vi "App - analyze RUS V6.vi"() -> ()   [LabVIEW 2015] (continued)
oling_2nd_try/September_2014/091714/39.66500K_500_2500_2.10000V_0.00000T_Sep17-2014__15-02-56_001_091714.bin", "last mod"=timestamp(3493825376 s since 1904-01-01), "file name str"="D:\\Data\\Ultrasound\\LSCO\\LSCO22__130814c\\5_Cooling_2nd_try\\September_2014\\091714\\39.66500K_500_2500_2.10000V_0.00000T_Sep17-2014__15-02-56_001_091714.bin", "mod time(min)"=58230422.93333333, "file format"=enum."binary", "power(V)"=2.1, "Magn Field(T) "=0.0}, {"temperature"=39.59, "temperature str"="39.59000", "file path"=path "D:/Data/Ultrasound/LSCO/LSCO22__130814c/5_Cooling_2nd_try/September_2014/091714/39.59000K_500_2500_2.10000V_0.00000T_Sep17-2014__15-04-15_001_091714.bin", "last mod"=timestamp(3493825455 s since 1904-01-01), "file name str"="D:\\Data\\Ultrasound\\LSCO\\LSCO22__130814c\\5_Cooling_2nd_try\\September_2014\\091714\\39.59000K_500_2500_2.10000V_0.00000T_Sep17-2014__15-04-15_001_091714.bin", "mod time(min)"=58230424.25, "file format"=enum."binary", "power(V)"=2.1, "Magn Field(T) "=0.0}, {"temperature"=39.502, "temperature str"="39.50200", "file path"=path "D:/Data/Ultrasound/LSCO/LSCO22__130814c/5_Cooling_2nd_try/September_2014/091714/39.50200K_500_2500_2.10000V_0.00000T_Sep17-2014__15-05-35_001_091714.bin", "last mod"=timestamp(3493825535 s since 1904-01-01), "file name str"="D:\\Data\\Ultrasound\\LSCO\\LSCO22__130814c\\5_Cooling_2nd_try\\September_2014\\091714\\39.50200K_500_2500_2.10000V_0.00000T_Sep17-2014__15-05-35_001_091714.bin", "mod time(min)"=58230425.583333336, "file format"=enum."binary", "power(V)"=2.1, "Magn Field(T) "=0.0}, {"temperature"=39.427, "temperature str"="39.42700", "file path"=path "D:/Data/Ultrasound/LSCO/LSCO22__130814c/5_Cooling_2nd_try/September_2014/091714/39.42700K_500_2500_2.10000V_0.00000T_Sep17-2014__15-06-54_001_091714.bin", "last mod"=timestamp(3493825614 s since 1904-01-01), "file name str"="D:\\Data\\Ultrasound\\LSCO\\LSCO22__130814c\\5_Cooling_2nd_try\\September_2014\\091714\\39.42700K_500_2500_2.10000V_0.00000T_Sep17-2014__15-06-54_001_091714.bin", "mod time(min)"=58230426.9, "file format"=enum."binary", "power(V)"=2.1, "Magn Field(T) "=0.0}, {"temperature"=39.345, "temperature str"="39.34500", "file path"=path "D:/Data/Ultrasound/LSCO/LSCO22__130814c/5_Cooling_2nd_try/September_2014/091714/39.34500K_500_2500_2.10000V_0.00000T_Sep17-2014__15-08-13_001_091714.bin", "last mod"=timestamp(3493825693 s since 1904-01-01), "file name str"="D:\\Data\\Ultrasound\\LSCO\\LSCO22__130814c\\5_Cooling_2nd_try\\September_2014\\091714\\39.34500K_500_2500_2.10000V_0.00000T_Sep17-2014__15-08-13_001_091714.bin", "mod time(min)"=58230428.21666667, "file format"=enum."binary", "power(V)"=2.1, "Magn Field(T) "=0.0}, {"temperature"=39.266, "temperature str"="39.26600", "file path"=path "D:/Data/Ultrasound/LSCO/LSCO22__130814c/5_Cooling_2nd_try/September_2014/091714/39.26600K_500_2500_2.10000V_0.00000T_Sep17-2014__15-09-33_001_091714.bin", "last mod"=timestamp(3493825773 s since 1904-01-01), "file name str"="D:\\Data\\Ultrasound\\LSCO\\LSCO22__130814c\\5_Cooling_2nd_try\\September_2014\\091714\\39.26600K_500_2500_2.10000V_0.00000T_Sep17-2014__15-09-33_001_091714.bin", "mod time(min)"=58230429.55, "file format"=enum."binary", "power(V)"=2.1, "Magn Field(T) "=0.0}, {"temperature"=39.182, "temperature str"="39.18200", "file path"=path "D:/Data/Ultrasound/LSCO/LSCO22__130814c/5_Cooling_2nd_try/September_2014/091714/39.18200K_500_2500_2.10000V_0.00000T_Sep17-2014__15-10-52_001_091714.bin", "last mod"=timestamp(3493825852 s since 1904-01-01), "file name str"="D:\\Data\\Ultrasound\\LSCO\\LSCO22__130814c\\5_Cooling_2nd_try\\September_2014\\091714\\39.18200K_500_2500_2.10000V_0.00000T_Sep17-2014__15-10-52_001_091714.bin", "mod time(min)"=58230430.86666667, "file format"=enum."binary", "power(V)"=2.1, "Magn Field(T) "=0.0}, {"temperature"=39.106, "temperature str"="39.10600", "file path"=path "D:/Data/Ultrasound/LSCO/LSCO22__130814c/5_Cooling_2nd_try/September_2014/091714/39.10600K_500_2500_2.10000V_0.00000T_Sep17-2014__15-12-11_001_091714.bin", "last mod"=timestamp(3493825931 s since 1904-01-01), "file name str"="D:\\Data\\Ultrasound\\LSCO\\LSCO22__130814c\\5_Cooling_2nd_try\\September_2014\\091714\\39.10600K_500_2500_2.10000V_0.00000T_Sep17-2014__15-12-11_001_091714.bin", "mod time(min)"=58230432.18333333, "file format"=enum."binary", "power(V)"=2.1, "Magn Field(T) "=0.0}, {"temperature"=39.022, "temperature str"="39.02200", "file path"=path "D:/Data/Ultrasound/LSCO/LSCO22__130814c/5_Cooling_2nd_try/September_2014/091714/39.02200K_500_2500_2.10000V_0.00000T_Sep17-2014__15-13-31_001_091714.bin", "last mod"=timestamp(3493826011 s since 1904-01-01), "file name str"="D:\\Data\\Ultrasound\\LSCO\\LSCO22__130814c\\5_Cooling_2nd_try\\September_2014\\091714\\39.02200K_500_2500_2.10000V_0.00000T_Sep17-2014__15-13-31_001_091714.bin", "mod time(min)"=58230433.516666666, "file format"=enum."binary", "power(V)"=2.1, "Magn Field(T) "=0.0}, {"temperature"=38.943, "temperature str"="38.94300", "file path"=path "D:/Data/Ultrasound/LSCO/LSCO22__130814c/5_Cooling_2nd_try/September_2014/091714/38.94300K_500_2500_2.10000V_0.00000T_Sep17-2014__15-14-50_001_091714.bin", "last mod"=timestamp(3493826090 s since 1904-01-01), "file name str"="D:\\Data\\Ultrasound\\LSCO\\LSCO22__130814c\\5_Cooling_2nd_try\\September_2014\\091714\\38.94300K_500_2500_2.10000V_0.00000T_Sep17-2014__15-14-50_001_091714.bin", "mod time(min)"=58230434.833333336, "file format"=enum."binary", "power(V)"=2.1, "Magn Field(T) "=0.0}, {"temperature"=38.864, "temperature str"="38.86400", "file path"=path "D:/Data/Ultrasound/LSCO/LSCO22__130814c/5_Cooling_2nd_try/September_2014/091714/38.86400K_500_2500_2.10000V_0.00000T_Sep17-2014__15-16-10_001_091714.bin", "last mod"=timestamp(3493826170 s since 1904-01-01), "file name str"="D:\\Data\\Ultrasound\\LSCO\\LSCO22__130814c\\5_Cooling_2nd_try\\September_2014\\091714\\38.86400K_500_2500_2.10000V_0.00000T_Sep17-2014__15-16-10_001_091714.bin", "mod time(min)"=58230436.166666664, "file format"=enum."binary", "power(V)"=2.1, "Magn Field(T) "=0.0}, {"temperature"=38.78, "temperature str"="38.78000", "file path"=path "D:/Data/Ultrasound/LSCO/LSCO22__130814c/5_Cooling_2nd_try/September_2014/091714/38.78000K_500_2500_2.10000V_0.00000T_Sep17-2014__15-17-29_001_091714.bin", "last mod"=timestamp(3493826249 s since 1904-01-01), "file name str"="D:\\Data\\Ultrasound\\LSCO\\LSCO22__130814c\\5_Cooling_2nd_try\\September_2014\\091714\\38.78000K_500_2500_2.10000V_0.00000T_Sep17-2014__15-17-29_001_091714.bin", "mod time(min)"=58230437.483333334, "file format"=enum."binary", "power(V)"=2.1, "Magn Field(T) "=0.0}, {"temperature"=38.695, "temperature str"="38.69500", "file path"=path "D:/Data/Ultrasound/LSCO/LSCO22__130814c/5_Cooling_2nd_try/September_2014/091714/38.69500K_500_2500_2.10000V_0.00000T_Sep17-2014__15-18-49_001_091714.bin", "last mod"=timestamp(3493826329 s since 1904-01-01), "file name str"="D:\\Data\\Ultrasound\\LSCO\\LSCO22__130814c\\5_Cooling_2nd_try\\September_2014\\091714\\38.69500K_500_2500_2.10000V_0.00000T_Sep17-2014__15-18-49_001_091714.bin", "mod time(min)"=58230438.81666667, "file format"=enum."binary", "power(V)"=2.1, "Magn Field(T) "=0.0}, {"temperature"=38.618, "temperature str"="38.61800", "file path"=path "D:/Data/Ultrasound/LSCO/LSCO22__130814c/5_Cooling_2nd_try/September_2014/091714/38.61800K_500_2500_2.10000V_0.00000T_Sep17-2014__15-20-08_001_091714.bin", "last mod"=timestamp(3493826408 s since 1904-01-01), "file name str"="D:\\Data\\Ultrasound\\LSCO\\LSCO22__130814c\\5_Cooling_2nd_try\\September_2014\\091714\\38.61800K_500_2500_2.10000V_0.00000T_Sep17-2014__15-20-08_001_091714.bin", "mod time(min)"=58230440.13333333, "file format"=enum."binary", "power(V)"=2.1, "Magn Field(T) "=0.0}, {"temperature"=38.531, "temperature str"="38.53100", "file path"=path "D:/Data/Ultrasound/LSCO/LSCO22__130814c/5_Cooling_2nd_try/September_2014/091714/38.53100K_500_2500_2.10000V_0.00000T_Sep17-2014__15-21-27_001_091714.bin", "last mod"=timestamp(3493826487 s since 1904-01-01), "file name str"="D:\\Data\\Ultrasound\\LSCO\\LSCO22__130814c\\5_Cooling_2nd_try\\September_2014\\091714\\38.53100K_500_2500_2.10000V_0.00000T_Sep17-2014__15-21-27_001_091714.bin", "mod time(min)"=58230441.45, "file format"=enum."binary", "power(V)"=2.1, "Magn Field(T) "=0.0}, {"temperature"=38.455, "temperature str"="38.45500", "file path"=path "D:/Data/Ultrasound/LSCO/LSCO22__130814c/5_Cooling_2nd_try/September_2014/091714/38.45500K_500_2500_2.10000V_0.00000T_Sep17-2014__15-22-47_001_091714.bin", "last mod"=timestamp(3493826567 s since 1904-01-01), "file name str"="D:\\Data\\Ultrasound\\LSCO\\LSCO22__130814c\\5_Cooling_2nd_try\\September_2014\\091714\\38.45500K_500_2500_2.10000V_0.00000T_Sep17-2014__15-22-47_001_091714.bin", "mod time(min)"=58230442.78333333, "file format"=enum."binary", "power(V)"=2.1, "Magn Field(T) "=0.0}, {"temperature"=38.37, "temperature str"="38.37000", "file path"=path "D:/Data/Ultrasound/LSCO/LSCO22__130814c/5_Cooling_2nd_try/September_2014/091714/38.37000K_500_2500_2.10000V_0.00000T_Sep17-2014__15-24-06_001_091714.bin", "last mod"=timestamp(3493826646 s since 1904-01-01), "file name str"="D:\\Data\\Ultrasound\\LSCO\\LSCO22__130814c\\5_Cooling_2nd_try\\September_2014\\091714\\38.37000K_500_2500_2.10000V_0.00000T_Sep17-2014__15-24-06_001_091714.bin", "mod time(min)"=58230444.1, "file format"=enum."binary", "power(V)"=2.1, "Magn Field(T) "=0.0}, {"temperature"=38.286, "temperature str"="38.28600", "file path"=path "D:/Data/Ultrasound/LSCO/LSCO22__130814c/5_Cooling_2nd_try/September_2014/091714/38.28600K_500_2500_2.10000V_0.00000T_Sep17-2014__15-25-25_001_091714.bin", "last mod"=timestamp(3493826725 s since 1904-01-01), "file name str"="D:\\Data\\Ultrasound\\LSCO\\LSCO22__130814c\\5_Cooling_2nd_try\\September_2014\\091714\\38.28600K_500_2500_2.10000V_0.00000T_Sep17-2014__15-25-25_001_091714.bin", "mod time(min)"=58230445.416666664, "file format"=enum."binary", "power(V)"=2.1, "Magn Field(T) "=0.0}, {"temperature"=38.203, "temperature str"="38.20300", "file path"=path "D:/Data/Ultrasound/LSCO/LSCO22__130814c/5_Cooling_2nd_try/September_2014/091714/38.20300K_500_2500_2.10000V_0.00000T_Sep17-2014__15-26-45_001_091714.bin", "last mod"=timestamp(3493826805 s since 1904-01-01), "file name str"="D:\\Data\\Ultrasound\\LSCO\\LSCO22__130814c\\5_Cooling_2nd_try\\September_2014\\091714\\38.20300K_500_2500_2.10000V_0.00000T_Sep17-2014__15-26-45_001_091714.bin", "mod time(min)"=58230446.75, "file format"=enum."binary", "power(V)"=2.1, "Magn Field(T) "=0.0}, {"temperature"=38.122, "temperature str"="38.12200", "file path"=path "D:/Data/Ultrasound/LSCO/LSCO22__130814c/5_Cooling_2nd_try/September_2014/091714/38.12200K_500_2500_2.10000V_0.00000T_Sep17-2014__15-28-04_001_091714.bin", "last mod"=timestamp(3493826884 s since 1904-01-01), "file name str"="D:\\Data\\Ultrasound\\LSCO\\LSCO22__130814c\\5_Cooling_2nd_try\\September_2014\\091714\\38.12200K_500_2500_2.10000V_0.00000T_Sep17-2014__15-28-04_001_091714.bin", "mod time(min)"=58230448.06666667, "file format"=enum."binary", "power(V)"=2.1, "Magn Field(T) "=0.0}, {"temperature"=38.042, "temperature str"="38.04200", "file path"=path "D:/Data/Ultrasound/LSCO/LSCO22__130814c/5_Cooling_2nd_try/September_2014/091714/38.04200K_500_2500_2.10000V_0.00000T_Sep17-2014__15-29-24_001_091714.bin", "last mod"=timestamp(3493826964 s since 1904-01-01), "file name str"="D:\\Data\\Ultrasound\\LSCO\\LSCO22__130814c\\5_Cooling_2nd_try\\September_2014\\091714\\38.04200K_500_2500_2.10000V_0.00000T_Sep17-2014__15-29-24_001_091714.bin", "mod time(min)"=58230449.4, "file format"=enum."binary", "power(V)"=2.1, "Magn Field(T) "=0.0}, {"temperature"=37.958, "temperature str"="37.95800", "file path"=path "D:/Data/Ultrasound/LSCO/LSCO22__130814c/5_Cooling_2nd_try/September_2014/091714/37.95800K_500_2500_2.10000V_0.00000T_Sep17-2014__15-30-43_001_091714.bin", "last mod"=timestamp(3493827043 s since 1904-01-01), "file name str"="D:\\Data\\Ultrasound\\LSCO\\LSCO22__130814c\\5_Cooling_2nd_try\\September_2014\\091714\\37.95800K_500_2500_2.10000V_0.00000T_Sep17-2014__15-30-43_001_091714.bin", "mod time(min)"=58230450.71666667, "file format"=enum."binary", "power(V)"=2.1, "Magn Field(T) "=0.0}, {"temperature"=37.876, "temperature str"="37.87600", "file path"=path "D:/Data/Ultrasound/LSCO/LSCO22__130814c/5_Cooling_2nd_try/September_2014/091714/37.87600K_500_2500_2.10000V_0.00000T_Sep17-2014__15-32-02_001_091714.bin", "last mod"=timestamp(3493827122 s since 1904-01-01), "file name str"="D:\\Data\\Ultrasound\\LSCO\\LSCO22__130814c\\5_Cooling_2nd_try\\September_2014\\091714\\37.87600K_500_2500_2.10000V_0.00000T_Sep17-2014__15-32-02_001_091714.bin", "mod time(min)"=58230452.03333333, "file format"=enum."binary", "power(V)"=2.1, "Magn Field(T) "=0.0}, {"temperature"=37.797, "temperature str"="37.79700", "file path"=path "D:/Data/Ultrasound/LSCO/LSCO22__130814c/5_Cooling_2nd_try/September_2014/091714/37.79700K_500_2500_2.10000V_0.00000T_Sep17-2014__15-33-22_001_091714.bin", "last mod"=timestamp(3493827202 s since 1904-01-01), "file name str"="D:\\Data\\Ultrasound\\LSCO\\LSCO22__130814c\\5_Cooling_2nd_try\\September_2014\\091714\\37.79700K_500_2500_2.10000V_0.00000T_Sep17-2014__15-33-22_001_091714.bin", "mod time(min)"=58230453.36666667, "file format"=enum."binary", "power(V)"=2.1, "Magn Field(T) "=0.0}, {"temperature"=37.711, "temperature str"="37.71100", "file path"=path "D:/Data/Ultrasound/LSCO/LSCO22__130814c/5_Cooling_2nd_try/September_2014/091714/37.71100K_500_2500_2.10000V_0.00000T_Sep17-2014__15-34-41_001_091714.bin", "last mod"=timestamp(3493827281 s since 1904-01-01), "file name str"="D:\\Data\\Ultrasound\\LSCO\\LSCO22__130814c\\5_Cooling_2nd_try\\September_2014\\091714\\37.71100K_500_2500_2.10000V_0.00000T_Sep17-2014__15-34-41_001_091714.bin", "mod time(min)"=58230454.68333333, "file format"=enum."binary", "power(V)"=2.1, "Magn Field(T) "=0.0}, {"temperature"=37.627, "temperature str"="37.62700", "file path"=path "D:/Data/Ultrasound/LSCO/LSCO22__130814c/5_Cooling_2nd_try/September_2014/091714/37.62700K_500_2500_2.10000V_0.00000T_Sep17-2014__15-36-00_001_091714.bin", "last mod"=timestamp(3493827360 s since 1904-01-01), "file name str"="D:\\Data\\Ultrasound\\LSCO\\LSCO22__130814c\\5_Cooling_2nd_try\\September_2014\\091714\\37.62700K_500_2500_2.10000V_0.00000T_Sep17-2014__15-36-00_001_091714.bin", "mod time(min)"=58230456.0, "file format"=enum."binary", "power(V)"=2.1, "Magn Field(T) "=0.0}, {"temperature"=37.544, "temperature str"="37.54400", "file path"=path "D:/Data/Ultrasound/LSCO/LSCO22__130814c/5_Cooling_2nd_try/September_2014/091714/37.54400K_500_2500_2.10000V_0.00000T_Sep17-2014__15-37-20_001_091714.bin", "last mod"=timestamp(3493827440 s since 1904-01-01), "file name str"="D:\\Data\\Ultrasound\\LSCO\\LSCO22__130814c\\5_Cooling_2nd_try\\September_2014\\091714\\37.54400K_500_2500_2.10000V_0.00000T_Sep17-2014__15-37-20_001_091714.bin", "mod time(min)"=58230457.333333336, "file format"=enum."binary", "power(V)"=2.1, "Magn Field(T) "=0.0}, {"temperature"=37.459, "temperature str"="37.45900", "file path"=path "D:/Data/Ultrasound/LSCO/LSCO22__130814c/5_Cooling_2nd_try/September_2014/091714/37.45900K_500_2500_2.10000V_0.00000T_Sep17-2014__15-38-39_001_091714.bin", "last mod"=timestamp(3493827519 s since 1904-01-01), "file name str"="D:\\Data\\Ultrasound\\LSCO\\LSCO22__130814c\\5_Cooling_2nd_try\\September_2014\\091714\\37.45900K_500_2500_2.10000V_0.00000T_Sep17-2014__15-38-39_001_091714.bin", "mod time(min)"=58230458.65, "file format"=enum."binary", "power(V)"=2.1, "Magn Field(T) "=0.0}, {"temperature"=37.378, "temperature str"="37.37800", "file path"=path "D:/Data/Ultrasound/LSCO/LSCO22__130814c/5_Cooling_2nd_try/September_2014/091714/37.37800K_500_2500_2.10000V_0.00000T_Sep17-2014__15-39-59_001_091714.bin", "last mod"=timestamp(3493827599 s since 1904-01-01), "file name str"="D:\\Data\\Ultrasound\\LSCO\\LSCO22__130814c\\5_Cooling_2nd_try\\September_2014\\091714\\37.37800K_500_2500_2.10000V_0.00000T_Sep17-2014__15-39-59_001_091714.bin", "mod time(min)"=58230459.983333334, "file format"=enum."binary", "power(V)"=2.1, "Magn Field(T) "=0.0}, {"temperature"=37.297, "temperature str"="37.29700", "file path"=path "D:/Data/Ultrasound/LSCO/LSCO22__130814c/5_Cooling_2nd_try/September_2014/091714/37.29700K_500_2500_2.10000V_0.00000T_Sep17-2014__15-41-18_001_091714.bin", "last mod"=timestamp(3493827678 s since 1904-01-01), "file name str"="D:\\Data\\Ultrasound\\LSCO\\LSCO22__130814c\\5_Cooling_2nd_try\\September_2014\\091714\\37.29700K_500_2500_2.10000V_0.00000T_Sep17-2014__15-41-18_001_091714.bin", "mod time(min)"=58230461.3, "file format"=enum."binary", "power(V)"=2.1, "Magn Field(T) "=0.0}, {"temperature"=37.206, "temperature str"="37.20600", "file path"=path "D:/Data/Ultrasound/LSCO/LSCO22__130814c/5_Cooling_2nd_try/September_2014/091714/37.20600K_500_2500_2.10000V_0.00000T_Sep17-2014__15-42-37_001_091714.bin", "last mod"=timestamp(3493827757 s since 1904-01-01), "file name str"="D:\\Data\\Ultrasound\\LSCO\\LSCO22__130814c\\5_Cooling_2nd_try\\September_2014\\091714\\37.20600K_500_2500_2.10000V_0.00000T_Sep17-2014__15-42-37_001_091714.bin", "mod time(min)"=58230462.61666667, "file format"=enum."binary", "power(V)"=2.1, "Magn Field(T) "=0.0}, {"temperature"=37.129, "temperature str"="37.12900", "file path"=path "D:/Data/Ultrasound/LSCO/LSCO22__130814c/5_Cooling_2nd_try/September_2014/091714/37.12900K_500_2500_2.10000V_0.00000T_Sep17-2014__15-43-57_001_091714.bin", "last mod"=timestamp(3493827837 s since 1904-01-01), "file name str"="D:\\Data\\Ultrasound\\LSCO\\LSCO22__130814c\\5_Cooling_2nd_try\\September_2014\\091714\\37.12900K_500_2500_2.10000V_0.00000T_Sep17-2014__15-43-57_001_091714.bin", "mod time(min)"=58230463.95, "file format"=enum."binary", "power(V)"=2.1, "Magn Field(T) "=0.0}, {"temperature"=37.038, "temperature str"="37.03800", "file path"=path "D:/Data/Ultrasound/LSCO/LSCO22__130814c/5_Cooling_2nd_try/September_2014/091714/37.03800K_500_2500_2.10000V_0.00000T_Sep17-2014__15-45-16_001_091714.bin", "last mod"=timestamp(3493827916 s since 1904-01-01), "file name str"="D:\\Data\\Ultrasound\\LSCO\\LSCO22__130814c\\5_Cooling_2nd_try\\September_2014\\091714\\37.03800K_500_2500_2.10000V_0.00000T_Sep17-2014__15-45-16_001_091714.bin", "mod time(min)"=58230465.266666666, "file format"=enum."binary", "power(V)"=2.1, "Magn Field(T) "=0.0}, {"temperature"=36.964, "temperature str"="36.96400", "file path"=path "D:/Data/Ultrasound/LSCO/LSCO22__130814c/5_Cooling_2nd_try/September_2014/091714/36.96400K_500_2500_2.10000V_0.00000T_Sep17-2014__15-46-35_001_091714.bin", "last mod"=timestamp(3493827995 s since 1904-01-01), "file name str"="D:\\Data\\Ultrasound\\LSCO\\LSCO22__130814c\\5_Cooling_2nd_try\\September_2014\\091714\\36.96400K_500_2500_2.10000V_0.00000T_Sep17-2014__15-46-35_001_091714.bin", "mod time(min)"=58230466.583333336, "file format"=enum."binary", "power(V)"=2.1, "Magn Field(T) "=0.0}, {"temperature"=36.875, "temperature str"="36.87500", "file path"=path "D:/Data/Ultrasound/LSCO/LSCO22__130814c/5_Cooling_2nd_try/September_2014/091714/36.87500K_500_2500_2.10000V_0.00000T_Sep17-2014__15-47-55_001_091714.bin", "last mod"=timestamp(3493828075 s since 1904-01-01), "file name str"="D:\\Data\\Ultrasound\\LSCO\\LSCO22__130814c\\5_Cooling_2nd_try\\September_2014\\091714\\36.87500K_500_2500_2.10000V_0.00000T_Sep17-2014__15-47-55_001_091714.bin", "mod time(min)"=58230467.916666664, "file format"=enum."binary", "power(V)"=2.1, "Magn Field(T) "=0.0}, {"temperature"=36.787, "temperature str"="36.78700", "file path"=path "D:/Data/Ultrasound/LSCO/LSCO22__130814c/5_Cooling_2nd_try/September_2014/091714/36.78700K_500_2500_2.10000V_0.00000T_Sep17-2014__15-49-14_001_091714.bin", "last mod"=timestamp(3493828154 s since 1904-01-01), "file name str"="D:\\Data\\Ultrasound\\LSCO\\LSCO22__130814c\\5_Cooling_2nd_try\\September_2014\\091714\\36.78700K_500_2500_2.10000V_0.00000T_Sep17-2014__15-49-14_001_091714.bin", "mod time(min)"=58230469.233333334, "file format"=enum."binary", "power(V)"=2.1, "Magn Field(T) "=0.0}, {"temperature"=36.71, "temperature str"="36.71000", "file path"=path "D:/Data/Ultrasound/LSCO/LSCO22__130814c/5_Cooling_2nd_try/September_2014/091714/36.71000K_500_2500_2.10000V_0.00000T_Sep17-2014__15-50-34_001_091714.bin", "last mod"=timestamp(3493828234 s since 1904-01-01), "file name str"="D:\\Data\\Ultrasound\\LSCO\\LSCO22__130814c\\5_Cooling_2nd_try\\September_2014\\091714\\36.71000K_500_2500_2.10000V_0.00000T_Sep17-2014__15-50-34_001_091714.bin", "mod time(min)"=58230470.56666667, "file format"=enum."binary", "power(V)"=2.1, "Magn Field(T) "=0.0}, {"temperature"=36.616, "temperature str"="36.61600", "file path"=path "D:/Data/Ultrasound/LSCO/LSCO22__130814c/5_Cooling_2nd_try/September_2014/091714/36.61600K_500_2500_2.10000V_0.00000T_Sep17-2014__15-51-53_001_091714.bin", "last mod"=timestamp(3493828313 s since 1904-01-01), "file name str"="D:\\Data\\Ultrasound\\LSCO\\LSCO22__130814c\\5_Cooling_2nd_try\\September_2014\\091714\\36.61600K_500_2500_2.10000V_0.00000T_Sep17-2014__15-51-53_001_091714.bin", "mod time(min)"=58230471.88333333, "file format"=enum."binary", "power(V)"=2.1, "Magn Field(T) "=0.0}, {"temperature"=36.538, "temperature str"="36.53800", "file path"=path "D:/Data/Ultrasound/LSCO/LSCO22__130814c/5_Cooling_2nd_try/September_2014/091714/36.53800K_500_2500_2.10000V_0.00000T_Sep17-2014__15-53-12_001_091714.bin", "last mod"=timestamp(3493828392 s since 1904-01-01), "file name str"="D:\\Data\\Ultrasound\\LSCO\\LSCO22__130814c\\5_Cooling_2nd_try\\September_2014\\091714\\36.53800K_500_2500_2.10000V_0.00000T_Sep17-2014__15-53-12_001_091714.bin", "mod time(min)"=58230473.2, "file format"=enum."binary", "power(V)"=2.1, "Magn Field(T) "=0.0}, {"temperature"=36.457, "temperature str"="36.45700", "file path"=path "D:/Data/Ultrasound/LSCO/LSCO22__130814c/5_Cooling_2nd_try/September_2014/091714/36.45700K_500_2500_2.10000V_0.00000T_Sep17-2014__15-54-32_001_091714.bin", "last mod"=timestamp(3493828472 s since 1904-01-01), "file name str"="D:\\Data\\Ultrasound\\LSCO\\LSCO22__130814c\\5_Cooling_2nd_try\\September_2014\\091714\\36.45700K_500_2500_2.10000V_0.00000T_Sep17-2014__15-54-32_001_091714.bin", "mod time(min)"=58230474.53333333, "file format"=enum."binary", "power(V)"=2.1, "Magn Field(T) "=0.0}, {"temperature"=36.365, "temperature str"="36.36500", "file path"=path "D:/Data/Ultrasound/LSCO/LSCO22__130814c/5_Cooling_2nd_try/September_2014/091714/36.36500K_500_2500_2.10000V_0.00000T_Sep17-2014__15-55-51_001_091714.bin", "last mod"=timestamp(3493828551 s since 1904-01-01), "file name str"="D:\\Data\\Ultrasound\\LSCO\\LSCO22__130814c\\5_Cooling_2nd_try\\September_2014\\091714\\36.36500K_500_2500_2.10000V_0.00000T_Sep17-2014__15-55-51_001_091714.bin", "mod time(min)"=58230475.85, "file format"=enum."binary", "power(V)"=2.1, "Magn Field(T) "=0.0}, {"temperature"=36.288, "temperature str"="36.28800", "file path"=path "D:/Data/Ultrasound/LSCO/LSCO22__130814c/5_Cooling_2nd_try/September_2014/091714/36.28800K_500_2500_2.10000V_0.00000T_Sep17-2014__15-57-11_001_091714.bin", "last mod"=timestamp(3493828631 s since 1904-01-01), "file name str"="D:\\Data\\Ultrasound\\LSCO\\LSCO22__130814c\\5_Cooling_2nd_try\\September_2014\\091714\\36.28800K_500_2500_2.10000V_0.00000T_Sep17-2014__15-57-11_001_091714.bin", "mod time(min)"=58230477.18333333, "file format"=enum."binary", "power(V)"=2.1, "Magn Field(T) "=0.0}, {"temperature"=36.202, "temperature str"="36.20200", "file path"=path "D:/Data/Ultrasound/LSCO/LSCO22__130814c/5_Cooling_2nd_try/September_2014/091714/36.20200K_500_2500_2.10000V_0.00000T_Sep17-2014__15-58-30_001_091714.bin", "last mod"=timestamp(3493828710 s since 1904-01-01), "file name str"="D:\\Data\\Ultrasound\\LSCO\\LSCO22__130814c\\5_Cooling_2nd_try\\September_2014\\091714\\36.20200K_500_2500_2.10000V_0.00000T_Sep17-2014__15-58-30_001_091714.bin", "mod time(min)"=58230478.5, "file format"=enum."binary", "power(V)"=2.1, "Magn Field(T) "=0.0}, {"temperature"=36.116, "temperature str"="36.11600", "file path"=path "D:/Data/Ultrasound/LSCO/LSCO22__130814c/5_Cooling_2nd_try/September_2014/091714/36.11600K_500_2500_2.10000V_0.00000T_Sep17-2014__15-59-49_001_091714.bin", "last mod"=timestamp(3493828789 s since 1904-01-01), "file name str"="D:\\Data\\Ultrasound\\LSCO\\LSCO22__130814c\\5_Cooling_2nd_try\\September_2014\\091714\\36.11600K_500_2500_2.10000V_0.00000T_Sep17-2014__15-59-49_001_091714.bin", "mod time(min)"=58230479.81666667, "file format"=enum."binary", "power(V)"=2.1, "Magn Field(T) "=0.0}, {"temperature"=36.028, "temperature str"="36.02800", "file path"=path "D:/Data/Ultrasound/LSCO/LSCO22__130814c/5_Cooling_2nd_try/September_2014/091714/36.02800K_500_2500_2.10000V_0.00000T_Sep17-2014__16-01-09_001_091714.bin", "last mod"=timestamp(3493828869 s since 1904-01-01), "file name str"="D:\\Data\\Ultrasound\\LSCO\\LSCO22__130814c\\5_Cooling_2nd_try\\September_2014\\091714\\36.02800K_500_2500_2.10000V_0.00000T_Sep17-2014__16-01-09_001_091714.bin", "mod time(min)"=58230481.15, "file format"=enum."binary", "power(V)"=2.1, "Magn Field(T) "=0.0}, {"temperature"=35.946, "temperature str"="35.94600", "file path"=path "D:/Data/Ultrasound/LSCO/LSCO22__130814c/5_Cooling_2nd_try/September_2014/091714/35.94600K_500_2500_2.10000V_0.00000T_Sep17-2014__16-02-28_001_091714.bin", "last mod"=timestamp(3493828948 s since 1904-01-01), "file name str"="D:\\Data\\Ultrasound\\LSCO\\LSCO22__130814c\\5_Cooling_2nd_try\\September_2014\\091714\\35.94600K_500_2500_2.10000V_0.00000T_Sep17-2014__16-02-28_001_091714.bin", "mod time(min)"=58230482.46666667, "file format"=enum."binary", "power(V)"=2.1, "Magn Field(T) "=0.0}, {"temperature"=35.859, "temperature str"="35.85900", "file path"=path "D:/Data/Ultrasound/LSCO/LSCO22__130814c/5_Cooling_2nd_try/September_2014/091714/35.85900K_500_2500_2.10000V_0.00000T_Sep17-2014__16-03-47_001_091714.bin", "last mod"=timestamp(3493829027 s since 1904-01-01), "file name str"="D:\\Data\\Ultrasound\\LSCO\\LSCO22__130814c\\5_Cooling_2nd_try\\September_2014\\091714\\35.85900K_500_2500_2.10000V_0.00000T_Sep17-2014__16-03-47_001_091714.bin", "mod time(min)"=58230483.78333333, "file format"=enum."binary", "power(V)"=2.1, "Magn Field(T) "=0.0}, {"temperature"=35.776, "temperature str"="35.77600", "file path"=path "D:/Data/Ultrasound/LSCO/LSCO22__130814c/5_Cooling_2nd_try/September_2014/091714/35.77600K_500_2500_2.10000V_0.00000T_Sep17-2014__16-05-07_001_091714.bin", "last mod"=timestamp(3493829107 s since 1904-01-01), "file name str"="D:\\Data\\Ultrasound\\LSCO\\LSCO22__130814c\\5_Cooling_2nd_try\\September_2014\\091714\\35.77600K_500_2500_2.10000V_0.00000T_Sep17-2014__16-05-07_001_091714.bin", "mod time(min)"=58230485.11666667, "file format"=enum."binary", "power(V)"=2.1, "Magn Field(T) "=0.0}, {"temperature"=35.691, "temperature str"="35.69100", "file path"=path "D:/Data/Ultrasound/LSCO/LSCO22__130814c/5_Cooling_2nd_try/September_2014/091714/35.69100K_500_2500_2.10000V_0.00000T_Sep17-2014__16-06-26_001_091714.bin", "last mod"=timestamp(3493829186 s since 1904-01-01), "file name str"="D:\\Data\\Ultrasound\\LSCO\\LSCO22__130814c\\5_Cooling_2nd_try\\September_2014\\091714\\35.69100K_500_2500_2.10000V_0.00000T_Sep17-2014__16-06-26_001_091714.bin", "mod time(min)"=58230486.43333333, "file format"=enum."binary", "power(V)"=2.1, "Magn Field(T) "=0.0}, {"temperature"=35.608, "temperature str"="35.60800", "file path"=path "D:/Data/Ultrasound/LSCO/LSCO22__130814c/5_Cooling_2nd_try/September_2014/091714/35.60800K_500_2500_2.10000V_0.00000T_Sep17-2014__16-07-46_001_091714.bin", "last mod"=timestamp(3493829266 s since 1904-01-01), "file name str"="D:\\Data\\Ultrasound\\LSCO\\LSCO22__130814c\\5_Cooling_2nd_try\\September_2014\\091714\\35.60800K_500_2500_2.10000V_0.00000T_Sep17-2014__16-07-46_001_091714.bin", "mod time(min)"=58230487.766666666, "file format"=enum."binary", "power(V)"=2.1, "Magn Field(T) "=0.0}, {"temperature"=35.519, "temperature str"="35.51900", "file path"=path "D:/Data/Ultrasound/LSCO/LSCO22__130814c/5_Cooling_2nd_try/September_2014/091714/35.51900K_500_2500_2.10000V_0.00000T_Sep17-2014__16-09-05_001_091714.bin", "last mod"=timestamp(3493829345 s since 1904-01-01), "file name str"="D:\\Data\\Ultrasound\\LSCO\\LSCO22__130814c\\5_Cooling_2nd_try\\September_2014\\091714\\35.51900K_500_2500_2.10000V_0.00000T_Sep17-2014__16-09-05_001_091714.bin", "mod time(min)"=58230489.083333336, "file format"=enum."binary", "power(V)"=2.1, "Magn Field(T) "=0.0}, {"temperature"=35.437, "temperature str"="35.43700", "file path"=path "D:/Data/Ultrasound/LSCO/LSCO22__130814c/5_Cooling_2nd_try/September_2014/091714/35.43700K_500_2500_2.10000V_0.00000T_Sep17-2014__16-10-24_001_091714.bin", "last mod"=timestamp(3493829424 s since 1904-01-01), "file name str"="D:\\Data\\Ultrasound\\LSCO\\LSCO22__130814c\\5_Cooling_2nd_try\\September_2014\\091714\\35.43700K_500_2500_2.10000V_0.00000T_Sep17-2014__16-10-24_001_091714.bin", "mod time(min)"=58230490.4, "file format"=enum."binary", "power(V)"=2.1, "Magn Field(T) "=0.0}, {"temperature"=35.349, "temperature str"="35.34900", "file path"=path "D:/Data/Ultrasound/LSCO/LSCO22__130814c/5_Cooling_2nd_try/September_2014/091714/35.34900K_500_2500_2.10000V_0.00000T_Sep17-2014__16-11-44_001_091714.bin", "last mod"=timestamp(3493829504 s since 1904-01-01), "file name str"="D:\\Data\\Ultrasound\\LSCO\\LSCO22__130814c\\5_Cooling_2nd_try\\September_2014\\091714\\35.34900K_500_2500_2.10000V_0.00000T_Sep17-2014__16-11-44_001_091714.bin", "mod time(min)"=58230491.733333334, "file format"=enum."binary", "power(V)"=2.1, "Magn Field(T) "=0.0}, {"temperature"=35.264, "temperature str"="35.26400", "file path"=path "D:/Data/Ultrasound/LSCO/LSCO22__130814c/5_Cooling_2nd_try/September_2014/091714/35.26400K_500_2500_2.10000V_0.00000T_Sep17-2014__16-13-03_001_091714.bin", "last mod"=timestamp(3493829583 s since 1904-01-01), "file name str"="D:\\Data\\Ultrasound\\LSCO\\LSCO22__130814c\\5_Cooling_2nd_try\\September_2014\\091714\\35.26400K_500_2500_2.10000V_0.00000T_Sep17-2014__16-13-03_001_091714.bin", "mod time(min)"=58230493.05, "file format"=enum."binary", "power(V)"=2.1, "Magn Field(T) "=0.0}, {"temperature"=35.178, "temperature str"="35.17800", "file path"=path "D:/Data/Ultrasound/LSCO/LSCO22__130814c/5_Cooling_2nd_try/September_2014/091714/35.17800K_500_2500_2.10000V_0.00000T_Sep17-2014__16-14-23_001_091714.bin", "last mod"=timestamp(3493829663 s since 1904-01-01), "file name str"="D:\\Data\\Ultrasound\\LSCO\\LSCO22__130814c\\5_Cooling_2nd_try\\September_2014\\091714\\35.17800K_500_2500_2.10000V_0.00000T_Sep17-2014__16-14-23_001_091714.bin", "mod time(min)"=58230494.38333333, "file format"=enum."binary", "power(V)"=2.1, "Magn Field(T) "=0.0}, {"temperature"=35.091, "temperature str"="35.09100", "file path"=path "D:/Data/Ultrasound/LSCO/LSCO22__130814c/5_Cooling_2nd_try/September_2014/091714/35.09100K_500_2500_2.10000V_0.00000T_Sep17-2014__16-15-42_001_091714.bin", "last mod"=timestamp(3493829742 s since 1904-01-01), "file name str"="D:\\Data\\Ultrasound\\LSCO\\LSCO22__130814c\\5_Cooling_2nd_try\\September_2014\\091714\\35.09100K_500_2500_2.10000V_0.00000T_Sep17-2014__16-15-42_001_091714.bin", "mod time(min)"=58230495.7, "file format"=enum."binary", "power(V)"=2.1, "Magn Field(T) "=0.0}, {"temperature"=35.004, "temperature str"="35.00400", "file path"=path "D:/Data/Ultrasound/LSCO/LSCO22__130814c/5_Cooling_2nd_try/September_2014/091714/35.00400K_500_2500_2.10000V_0.00000T_Sep17-2014__16-17-01_001_091714.bin", "last mod"=timestamp(3493829821 s since 1904-01-01), "file name str"="D:\\Data\\Ultrasound\\LSCO\\LSCO22__130814c\\5_Cooling_2nd_try\\September_2014\\091714\\35.00400K_500_2500_2.10000V_0.00000T_Sep17-2014__16-17-01_001_091714.bin", "mod time(min)"=58230497.016666666, "file format"=enum."binary", "power(V)"=2.1, "Magn Field(T) "=0.0}, {"temperature"=34.918, "temperature str"="34.91800", "file path"=path "D:/Data/Ultrasound/LSCO/LSCO22__130814c/5_Cooling_2nd_try/September_2014/091714/34.91800K_500_2500_2.10000V_0.00000T_Sep17-2014__16-18-21_001_091714.bin", "last mod"=timestamp(3493829901 s since 1904-01-01), "file name str"="D:\\Data\\Ultrasound\\LSCO\\LSCO22__130814c\\5_Cooling_2nd_try\\September_2014\\091714\\34.91800K_500_2500_2.10000V_0.00000T_Sep17-2014__16-18-21_001_091714.bin", "mod time(min)"=58230498.35, "file format"=enum."binary", "power(V)"=2.1, "Magn Field(T) "=0.0}, {"temperature"=34.836, "temperature str"="34.83600", "file path"=path "D:/Data/Ultrasound/LSCO/LSCO22__130814c/5_Cooling_2nd_try/September_2014/091714/34.83600K_500_2500_2.10000V_0.00000T_Sep17-2014__16-19-40_001_091714.bin", "last mod"=timestamp(3493829980 s since 1904-01-01), "file name str"="D:\\Data\\Ultrasound\\LSCO\\LSCO22__130814c\\5_Cooling_2nd_try\\September_2014\\091714\\34.83600K_500_2500_2.10000V_0.00000T_Sep17-2014__16-19-40_001_091714.bin", "mod time(min)"=58230499.666666664, "file format"=enum."binary", "power(V)"=2.1, "Magn Field(T) "=0.0}, {"temperature"=34.745, "temperature str"="34.74500", "file path"=path "D:/Data/Ultrasound/LSCO/LSCO22__130814c/5_Cooling_2nd_try/September_2014/091714/34.74500K_500_2500_2.10000V_0.00000T_Sep17-2014__16-20-59_001_091714.bin", "last mod"=timestamp(3493830059 s since 1904-01-01), "file name str"="D:\\Data\\Ultrasound\\LSCO\\LSCO22__130814c\\5_Cooling_2nd_try\\September_2014\\091714\\34.74500K_500_2500_2.10000V_0.00000T_Sep17-2014__16-20-59_001_091714.bin", "mod time(min)"=58230500.983333334, "file format"=enum."binary", "power(V)"=2.1, "Magn Field(T) "=0.0}, {"temperature"=34.657, "temperature str"="34.65700", "file path"=path "D:/Data/Ultrasound/LSCO/LSCO22__130814c/5_Cooling_2nd_try/September_2014/091714/34.65700K_500_2500_2.10000V_0.00000T_Sep17-2014__16-22-19_001_091714.bin", "last mod"=timestamp(3493830139 s since 1904-01-01), "file name str"="D:\\Data\\Ultrasound\\LSCO\\LSCO22__130814c\\5_Cooling_2nd_try\\September_2014\\091714\\34.65700K_500_2500_2.10000V_0.00000T_Sep17-2014__16-22-19_001_091714.bin", "mod time(min)"=58230502.31666667, "file format"=enum."binary", "power(V)"=2.1, "Magn Field(T) "=0.0}, {"temperature"=34.57, "temperature str"="34.57000", "file path"=path "D:/Data/Ultrasound/LSCO/LSCO22__130814c/5_Cooling_2nd_try/September_2014/091714/34.57000K_500_2500_2.10000V_0.00000T_Sep17-2014__16-23-38_001_091714.bin", "last mod"=timestamp(3493830218 s since 1904-01-01), "file name str"="D:\\Data\\Ultrasound\\LSCO\\LSCO22__130814c\\5_Cooling_2nd_try\\September_2014\\091714\\34.57000K_500_2500_2.10000V_0.00000T_Sep17-2014__16-23-38_001_091714.bin", "mod time(min)"=58230503.63333333, "file format"=enum."binary", "power(V)"=2.1, "Magn Field(T) "=0.0}, {"temperature"=34.486, "temperature str"="34.48600", "file path"=path "D:/Data/Ultrasound/LSCO/LSCO22__130814c/5_Cooling_2nd_try/September_2014/091714/34.48600K_500_2500_2.10000V_0.00000T_Sep17-2014__16-24-58_001_091714.bin", "last mod"=timestamp(3493830298 s since 1904-01-01), "file name str"="D:\\Data\\Ultrasound\\LSCO\\LSCO22__130814c\\5_Cooling_2nd_try\\September_2014\\091714\\34.48600K_500_2500_2.10000V_0.00000T_Sep17-2014__16-24-58_001_091714.bin", "mod time(min)"=58230504.96666667, "file format"=enum."binary", "power(V)"=2.1, "Magn Field(T) "=0.0}, {"temperature"=34.396, "temperature str"="34.39600", "file path"=path "D:/Data/Ultrasound/LSCO/LSCO22__130814c/5_Cooling_2nd_try/September_2014/091714/34.39600K_500_2500_2.10000V_0.00000T_Sep17-2014__16-26-17_001_091714.bin", "last mod"=timestamp(3493830377 s since 1904-01-01), "file name str"="D:\\Data\\Ultrasound\\LSCO\\LSCO22__130814c\\5_Cooling_2nd_try\\September_2014\\091714\\34.39600K_500_2500_2.10000V_0.00000T_Sep17-2014__16-26-17_001_091714.bin", "mod time(min)"=58230506.28333333, "file format"=enum."binary", "power(V)"=2.1, "Magn Field(T) "=0.0}, {"temperature"=34.305, "temperature str"="34.30500", "file path"=path "D:/Data/Ultrasound/LSCO/LSCO22__130814c/5_Cooling_2nd_try/September_2014/091714/34.30500K_500_2500_2.10000V_0.00000T_Sep17-2014__16-27-36_001_091714.bin", "last mod"=timestamp(3493830456 s since 1904-01-01), "file name str"="D:\\Data\\Ultrasound\\LSCO\\LSCO22__130814c\\5_Cooling_2nd_try\\September_2014\\091714\\34.30500K_500_2500_2.10000V_0.00000T_Sep17-2014__16-27-36_001_091714.bin", "mod time(min)"=58230507.6, "file format"=enum."binary", "power(V)"=2.1, "Magn Field(T) "=0.0}, {"temperature"=34.228, "temperature str"="34.22800", "file path"=path "D:/Data/Ultrasound/LSCO/LSCO22__130814c/5_Cooling_2nd_try/September_2014/091714/34.22800K_500_2500_2.10000V_0.00000T_Sep17-2014__16-28-56_001_091714.bin", "last mod"=timestamp(3493830536 s since 1904-01-01), "file name str"="D:\\Data\\Ultrasound\\LSCO\\LSCO22__130814c\\5_Cooling_2nd_try\\September_2014\\091714\\34.22800K_500_2500_2.10000V_0.00000T_Sep17-2014__16-28-56_001_091714.bin", "mod time(min)"=58230508.93333333, "file format"=enum."binary", "power(V)"=2.1, "Magn Field(T) "=0.0}, {"temperature"=34.134, "temperature str"="34.13400", "file path"=path "D:/Data/Ultrasound/LSCO/LSCO22__130814c/5_Cooling_2nd_try/September_2014/091714/34.13400K_500_2500_2.10000V_0.00000T_Sep17-2014__16-30-15_001_091714.bin", "last mod"=timestamp(3493830615 s since 1904-01-01), "file name str"="D:\\Data\\Ultrasound\\LSCO\\LSCO22__130814c\\5_Cooling_2nd_try\\September_2014\\091714\\34.13400K_500_2500_2.10000V_0.00000T_Sep17-2014__16-30-15_001_091714.bin", "mod time(min)"=58230510.25, "file format"=enum."binary", "power(V)"=2.1, "Magn Field(T) "=0.0}, {"temperature"=34.046, "temperature str"="34.04600", "file path"=path "D:/Data/Ultrasound/LSCO/LSCO22__130814c/5_Cooling_2nd_try/September_2014/091714/34.04600K_500_2500_2.10000V_0.00000T_Sep17-2014__16-31-34_001_091714.bin", "last mod"=timestamp(3493830694 s since 1904-01-01), "file name str"="D:\\Data\\Ultrasound\\LSCO\\LSCO22__130814c\\5_Cooling_2nd_try\\September_2014\\091714\\34.04600K_500_2500_2.10000V_0.00000T_Sep17-2014__16-31-34_001_091714.bin", "mod time(min)"=58230511.56666667, "file format"=enum."binary", "power(V)"=2.1, "Magn Field(T) "=0.0}, {"temperature"=33.968, "temperature str"="33.96800", "file path"=path "D:/Data/Ultrasound/LSCO/LSCO22__130814c/5_Cooling_2nd_try/September_2014/091714/33.96800K_500_2500_2.10000V_0.00000T_Sep17-2014__16-32-54_001_091714.bin", "last mod"=timestamp(3493830774 s since 1904-01-01), "file name str"="D:\\Data\\Ultrasound\\LSCO\\LSCO22__130814c\\5_Cooling_2nd_try\\September_2014\\091714\\33.96800K_500_2500_2.10000V_0.00000T_Sep17-2014__16-32-54_001_091714.bin", "mod time(min)"=58230512.9, "file format"=enum."binary", "power(V)"=2.1, "Magn Field(T) "=0.0}, {"temperature"=33.87, "temperature str"="33.87000", "file path"=path "D:/Data/Ultrasound/LSCO/LSCO22__130814c/5_Cooling_2nd_try/September_2014/091714/33.87000K_500_2500_2.10000V_0.00000T_Sep17-2014__16-34-13_001_091714.bin", "last mod"=timestamp(3493830853 s since 1904-01-01), "file name str"="D:\\Data\\Ultrasound\\LSCO\\LSCO22__130814c\\5_Cooling_2nd_try\\September_2014\\091714\\33.87000K_500_2500_2.10000V_0.00000T_Sep17-2014__16-34-13_001_091714.bin", "mod time(min)"=58230514.21666667, "file format"=enum."binary", "power(V)"=2.1, "Magn Field(T) "=0.0}, {"temperature"=33.785, "temperature str"="33.78500", "file path"=path "D:/Data/Ultrasound/LSCO/LSCO22__130814c/5_Cooling_2nd_try/September_2014/091714/33.78500K_500_2500_2.10000V_0.00000T_Sep17-2014__16-35-33_001_091714.bin", "last mod"=timestamp(3493830933 s since 1904-01-01), "file name str"="D:\\Data\\Ultrasound\\LSCO\\LSCO22__130814c\\5_Cooling_2nd_try\\September_2014\\091714\\33.78500K_500_2500_2.10000V_0.00000T_Sep17-2014__16-35-33_001_091714.bin", "mod time(min)"=58230515.55, "file format"=enum."binary", "power(V)"=2.1, "Magn Field(T) "=0.0}, {"temperature"=33.699, "temperature str"="33.69900", "file path"=path "D:/Data/Ultrasound/LSCO/LSCO22__130814c/5_Cooling_2nd_try/September_2014/091714/33.69900K_500_2500_2.10000V_0.00000T_Sep17-2014__16-36-52_001_091714.bin", "last mod"=timestamp(3493831012 s since 1904-01-01), "file name str"="D:\\Data\\Ultrasound\\LSCO\\LSCO22__130814c\\5_Cooling_2nd_try\\September_2014\\091714\\33.69900K_500_2500_2.10000V_0.00000T_Sep17-2014__16-36-52_001_091714.bin", 
